vi "tc_init.vi"(0 "TC Label":string, 5 "Temperature":dbl format="%#_13g", 7 "Graph ON/OFF":u32(colorbox)=4250624, 9 "Plot Color":u32(colorbox)=16860, 11 "Alarm String":string, 12 "index (row)":i32, 13 "AlarmColor":u32(colorbox)) -> (4 "output array":T1(array[cluster]))   [LabVIEW 2017]
panel:
  in  "stop":bool
  in  "index (col)":i32
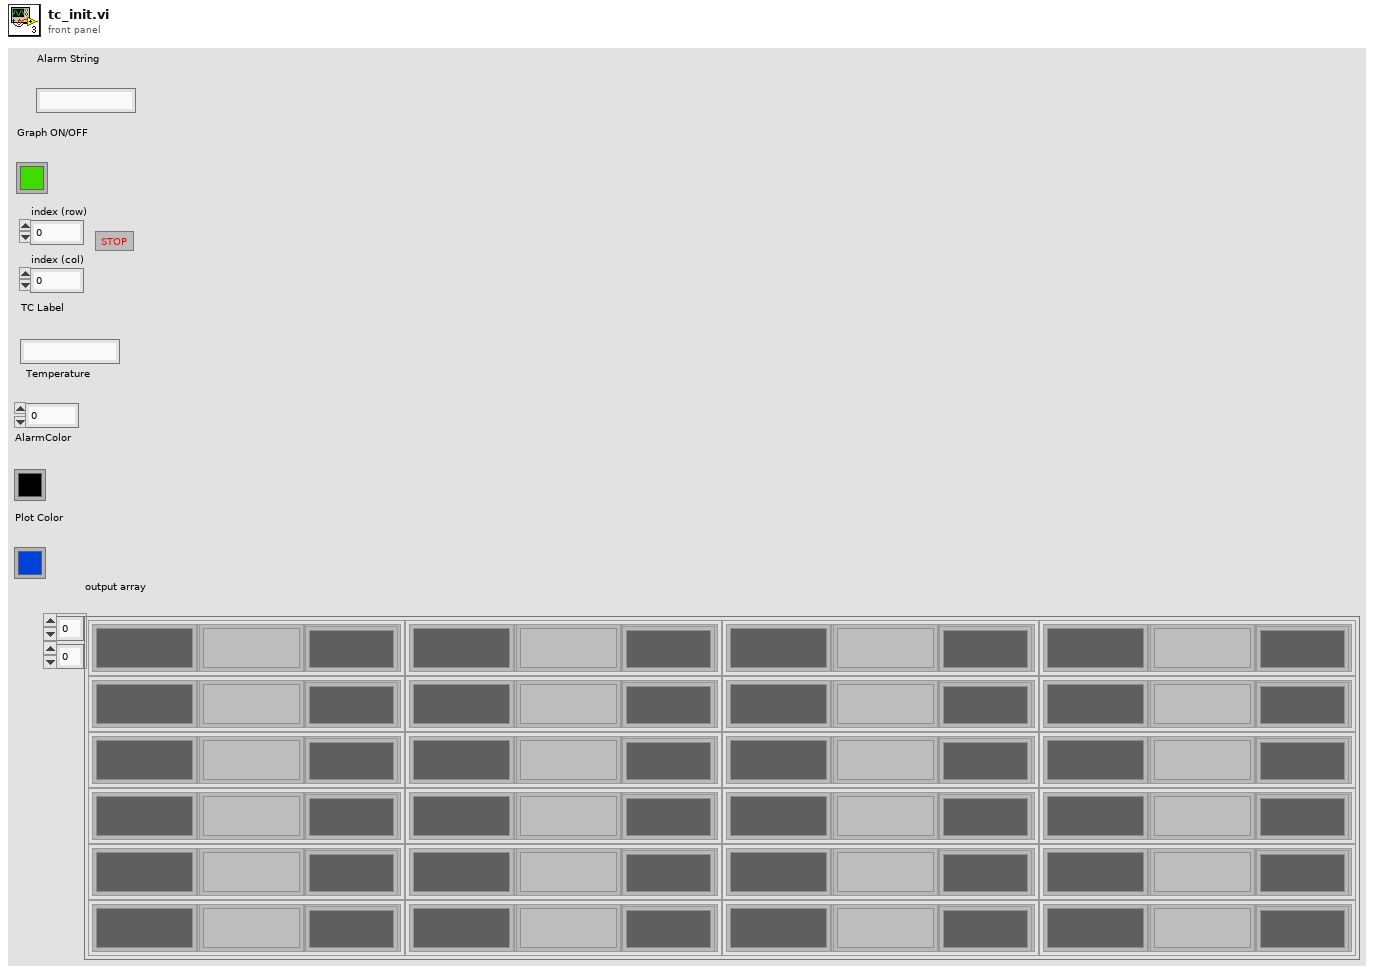
[diagram p1: front panel]
types:
  T1 = cluster{"TC Label":string, "Alarm Status":string, "Alarm Color":u32, "Temperature":string, "PlotColor":u32, "Graph On/Off":u32}[][]
  T2 = cluster{"TC Label":string, "Alarm Status":string, "Alarm Color":u32, "Temperature":string, "PlotColor":u32, "Graph On/Off":u32}
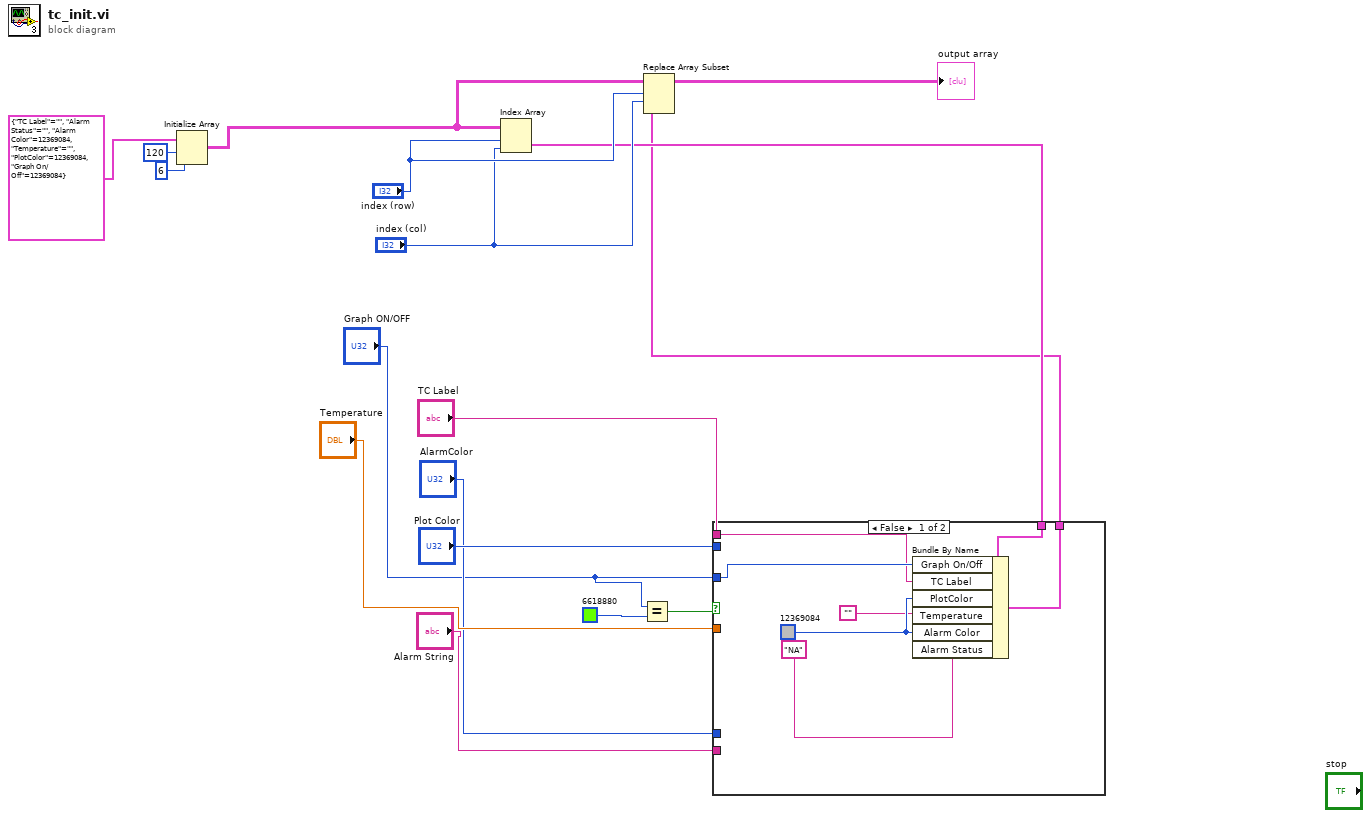
[diagram p0: block diagram]
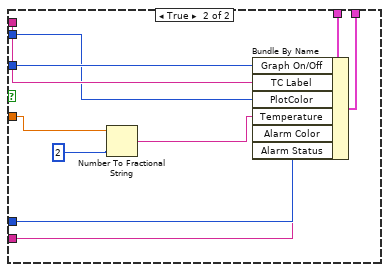
[diagram p2: hidden frame]
diagram:
  n1 = Initialize Array(T2 {"TC Label"="", "Alarm Status"="", "Alarm Color"=12369084, "Temperature"="", "PlotColor"=12369084, "Graph On/Off"=12369084}, 120 ("dimension size"), 6 ("dimension size")) -> (w15:T1)
  n2 = Index Array(array=w15, index (row)="index (row)", index (col)="index (col)") -> (element=w12:T2)
  n3 = Equal?(x="Graph ON/OFF", y=u32 6618880) -> (x = y?=w3:bool)
  n4 = case shown="False" w3 {
    tunnel: w12 -> [w24 w34]
    tunnel: "Graph ON/OFF" -> [w22 w33]
    tunnel: "TC Label" -> [w19 w32]
    tunnel: "Plot Color" -> [_ w31]
    tunnel: "Temperature" -> [_ w27]
    tunnel: "AlarmColor" -> [_ w30]
    tunnel: "Alarm String" -> [_ w29]
    tunnel: [w23 w28] -> w6
    frame False {
      w20 = u32 12369084 ("Alarm Color")
      n5 = Bundle By Name(cluster=w24, "Graph On/Off"=w22, "TC Label"=w19, "PlotColor"=w20, "Temperature"="", "Alarm Color"=w20, "Alarm Status"="NA") -> (w23:T2)
    }
    frame True {
      n6 = Number To Fractional String(number=w27, precision (6)=i16 2 ("width (-)")) -> (F-format string=w26:string)  [unwired: 2 in]
      n7 = Bundle By Name(cluster=w34, "Graph On/Off"=w33, "TC Label"=w32, "PlotColor"=w31, "Temperature"=w26, "Alarm Color"=w30, "Alarm Status"=w29) -> (w28:T2)
    }
  }
  n8 = Replace Array Subset(array=w15, new element=w6, index (row)="index (row)", index (col)="index (col)") -> (→"output array":T1)
